vi "CH_LM Config Units.vi"(0 "Meter Index":i32, 1 "Wavelength / nm":u32, 3 "Option (Value)":enum16{"MINIMUM", "Value", "MAXIMUM"}(ring)=enum."Value", 5 "error in (no error)":errorcluster, 7 "Timeout / ms (3000)":i32=1000, 8 "Action (query)":bool, 9 "Lock Timeout / ms (1000)":i32=1000) -> (11 "Lock timed out":bool, 14 "Meter Index":i32, 15 "Wavelength / nm":u32, 19 "error out":errorcluster)   [LabVIEW 2012, in "CH_LM.lvlib"]
doc: "This VI requests the LabMax to set and/or read the wavelength.\nOptionally the default wavelength can be read.\n\n<B>Note:</B> Request requires that a detector is connected.\n\n<B>Attention:</B>\nIf the requested wavelength is greater than the upper limit, the LabMax will set and return the upper wavelength limit. If the requested wavelength is less than the lower limit, the LabMax will set and return the lower wavelength limit."
uses:
  CH_LM.lvlib
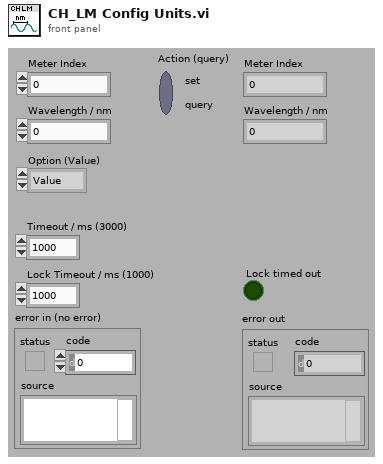
[diagram p1: front panel]
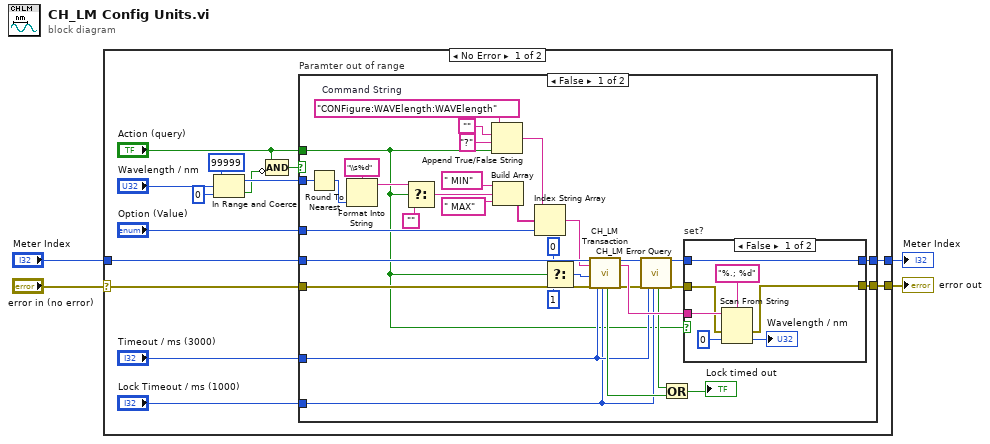
[diagram p0: block diagram]
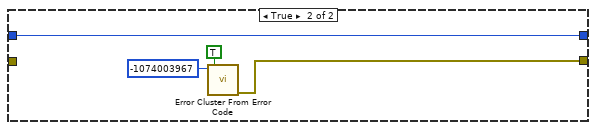
[diagram p3: hidden frame]
diagram:
  n1 = case shown="No Error" "error in (no error)" {
    selector: "error in (no error)" -> [w18 w66]
    tunnel: [w16 w66] -> w4
    tunnel: "Meter Index" -> [w17 w65]
    tunnel: [w14 w65] -> w1
    frame No Error {
      n2 = In Range and Coerce(upper limit=u32 99999, x="Wavelength / nm", lower limit=u32 0) -> (coerced(x)=w10:u32, In Range?=w7:bool)
      n3 = Compound Arithmetic op=AND("Action (query)", invert w7) -> (w5:bool)
      n4 = case "Paramter out of range" shown="False" w5 {
        tunnel: w18 -> [w51 _]
        tunnel: w17 -> [w50 w64]
        tunnel: [w47 w62] -> w16
        tunnel: "Option (Value)" -> [w40 _]
        tunnel: [w30 w64] -> w14
        tunnel: "Timeout / ms (3000)" -> [w22 _]
        tunnel: "Lock Timeout / ms (1000)" -> [w21 _]
        tunnel: w10 -> [w20 _]
        tunnel: "Action (query)" -> [w19 _]
        frame False {
          w49 = "CONFigure:WAVElength:WAVElength"  # Command String
          n5 = Round To Nearest(number=w20) -> (nearest integer value=w37:u32)
          n6 = Format Into String(format string="\\s%d", w37) -> (resulting string=w36:string)  [unwired: 2 in, 1 out]
          n7 = Select(t=w36, s=w19, f="") -> (s? t:f=w42:string)
          n8 = Append True/False String(1:w19, 2:"?" ("true string"), 3:"", 4:w49) -> (0:w39:string)
          n9 = Build Array(" MIN", w42, " MAX") -> (w38:string[])
          n10 = Index String Array(1:w40, 2:w38, 3:w39) -> (0:w34:string)
          n11 = Select(t=0, s=w19, f=1 ("NofStrings (-1:all)")) -> (s? t:f=w32:i32)
          n12 = call "CH_LM Transaction.vi"("Meter Index"=w50, "Command String"=w34, "NofStrings (-1:all)"=w32, "error in (no error)"=w51, "Timeout / ms (3000)"=w22, "Lock Timeout / ms (1000)"=w21) -> ("Lock timed out"=w24:bool, "Meter Index"=w29:i32, "Response"=w48:string, "error out"=w27:errorcluster)  [unwired: 10 out]
          n13 = call "CH_LM Error Query.vi"("Meter Index"=w29, "error in (no error)"=w27, "Timeout / ms (3000)"=w22, "Lock Timeout / ms (1000)"=w21) -> ("Lock timed out"=w25:bool, "Meter Index"=w28:i32, "error out"=w26:errorcluster)  [unwired: 13 out]
          n14 = Or(x=w25, y=w24) -> (x .or. y?=→"Lock timed out":bool)
          n15 = case "set?" shown="False" w19 {
            tunnel: w48 -> [w58 _]
            tunnel: w26 -> [w57 w60]
            tunnel: [w56 w60] -> w47
            tunnel: w28 -> [w52 w59]
            tunnel: [w52 w59] -> w30
            frame False {
              n16 = Scan From String(format string="%.; %d", input string=w58, error in=w57, default 1=u32 0 ("default value 1")) -> (error out=w56:errorcluster, output 1=→"Wavelength / nm":u32)  [unwired: 1 in, 2 out]
            }
            frame True {
            }
          }
        }
        frame True {
          n17 = call <vilib>:"Error Cluster From Error Code.vi"("show call chain? (False)"=TRUE, "error code (0)"=-1074003967) -> ("error out"=w62:errorcluster)  [unwired: 1 in, 6 out]
        }
      }
    }
    frame Error {
    }
  }
  "error out" <- w4
  "Meter Index" <- w1
